vi "load xml daq.vi"() -> ()   [LabVIEW 2013, in "DAQ.lvclass"]
uses:
  DAQ.lvclass
  <vilib>/Utility/xml.llb/Read From XML File(string).vi
panel:
  out "value":refnum<class "DAQ.lvclass">
  out "error out":errorcluster
  in  "error in (no error)":errorcluster
  in  "XML File Path":path
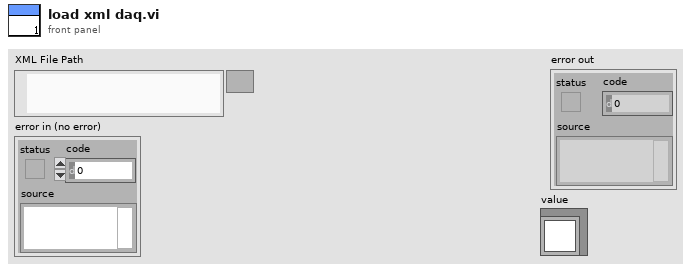
[diagram p1: front panel]
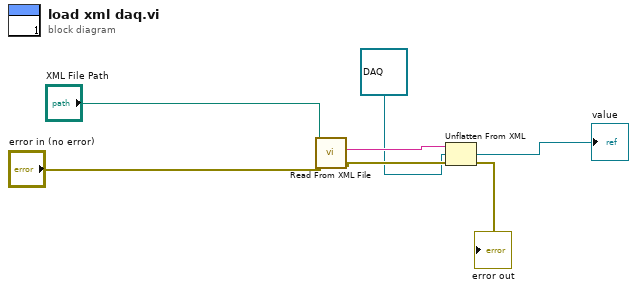
[diagram p0: block diagram]
diagram:
  n1 = call-poly <vilib>:"Read From XML File.vi"("error in (no error)"="error in (no error)", "XML File Path"="XML File Path") -> ("error out"=w4:errorcluster, "XML Elements"=w5:string)  [unwired: 7 in, 1 out]
  n2 = Unflatten From XML(xml string=w5, type=refnum<class "DAQ.lvclass"> refnum ("DAQ.lvclass"), error in (no error)=w4) -> (value=→"value":refnum<class "DAQ.lvclass">, error out=→"error out":errorcluster)
